vi "2526 Parse Scan List.vi"(10 "ApplicationNumberOfWeldChannels":i32=7, 11 "MUX Input String":string="SCANALL") -> (3 "Channel Array":string[](array[string])=["ch70", "ch71", "ch72", "ch73", "ch74", "ch75", "ch76"])   [LabVIEW 2019, in "SupportVIs.lvlib"]
uses:
  SupportVIs.lvlib
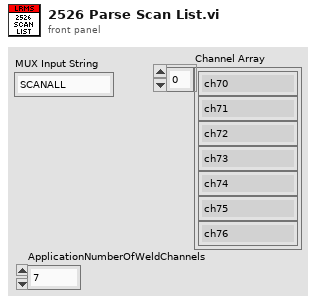
[diagram p1: front panel]
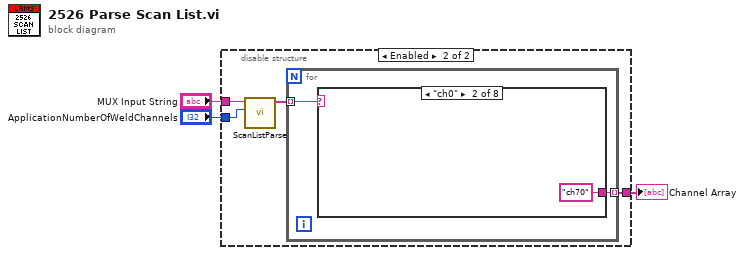
[diagram p0: block diagram]
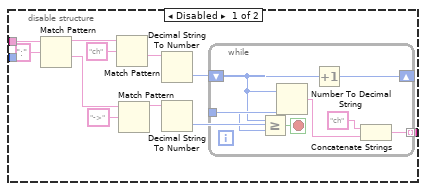
[diagram p2: hidden frame]
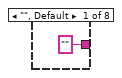
[diagram p3: hidden frame]
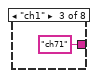
[diagram p4: hidden frame]
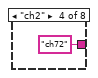
[diagram p5: hidden frame]
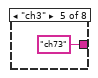
[diagram p6: hidden frame]
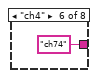
[diagram p7: hidden frame]
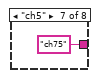
[diagram p8: hidden frame]
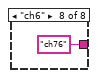
[diagram p9: hidden frame]
diagram:
  n1 = disable-structure shown="Enabled" {
    disable-tunnel: "MUX Input String" -> [w14 w25]
    disable-tunnel: [w4 w23] -> w2
    disable-tunnel: "ApplicationNumberOfWeldChannels" -> [_ w22]
    frame Disabled {
      n2 = Match Pattern(string=w14, regular expression=":" ("search string")) -> (before substring=w9:string, after substring=w12:string)  [unwired: 1 in, 2 out]
      n3 = Match Pattern(string=w9, regular expression="ch") -> (after substring=w8:string)  [unwired: 1 in, 3 out]
      n4 = Match Pattern(string=w12, regular expression="->") -> (before substring=w7:string)  [unwired: 1 in, 3 out]
      n5 = Decimal String To Number(string=w8) -> (number=w5:i32)  [unwired: 2 in, 1 out]
      n6 = Decimal String To Number(string=w7) -> (number=w6:i32)  [unwired: 2 in, 1 out]
      n7 = while {
        tunnel: w6 -> [w21]
        shift-right: [w19] -> _
        shift-left: w5 -> [w18]
        tunnel: [w15] -> w4 mode=indexing
        stop <- w20 stop-if-true
        n8 = Greater Or Equal?(x=w18, y=w21) -> (x >= y?=w20:bool)
        n9 = Number To Decimal String(number=w18) -> (decimal integer string=w16:string)  [unwired: 1 in]
        n10 = Increment(x=w18) -> (x+1=w19:i32)
        n11 = Concatenate Strings("ch" ("string"), w16) -> (w15:string)
      }
    }
    frame Enabled {
      n12 = call "ScanListParse.vi"("ApplicationNumberOfWeldChannels"=w22, "Input"=w25) -> ("Output"=w24:string[])  [unwired: 9 in]
      n13 = for {
        tunnel: w24 -> [w27] mode=indexing
        tunnel: [w26] -> w23 mode=indexing
        n14 = case shown="\"ch0\"" w27 {
          tunnel: ["" "ch70" "ch71" "ch72" "ch73" "ch74" "ch75" "ch76"] -> w26
          frame "", Default {
          }
          frame "ch0" {
          }
          frame "ch1" {
          }
          frame "ch2" {
          }
          frame "ch3" {
          }
          frame "ch4" {
          }
          frame "ch5" {
          }
          frame "ch6" {
          }
        }
      }
    }
  }
  "Channel Array" <- w2
